vi "_attribute_write_none.vi"(5 "Repeated Capability":string, 7 "Attribute":T1={"Identifier"="", "Descriptive Name"="", "Data Type"=enum."Integer 32", "Command"="", "Access"=enum."Read/Write", "Range Table"="", "Read Callback"="", "Write Callback"="", "Supported Models"="", "Instrument Options"="", "Index"=0, "OPC Wait"=FALSE, "No Status Check"=FALSE, "Cache Only"=FALSE}, 8 "error in":errorcluster caption="error in (no error)", 11 "VISA resource name":refnum<visa-resource-name>) -> (0 "error out":errorcluster, 3 "VISA resource name out":refnum<visa-resource-name>)   [LabVIEW 2020, in "Rohde&Schwarz RTx Oscilloscopes.lvlib" / "rsidr_core.lvlib"]
uses:
  rsidr_core.lvlib
  type_Attribute.ctl
  type_Attribute_Data_Type.ctl
  type_ReadWriteAccess.ctl
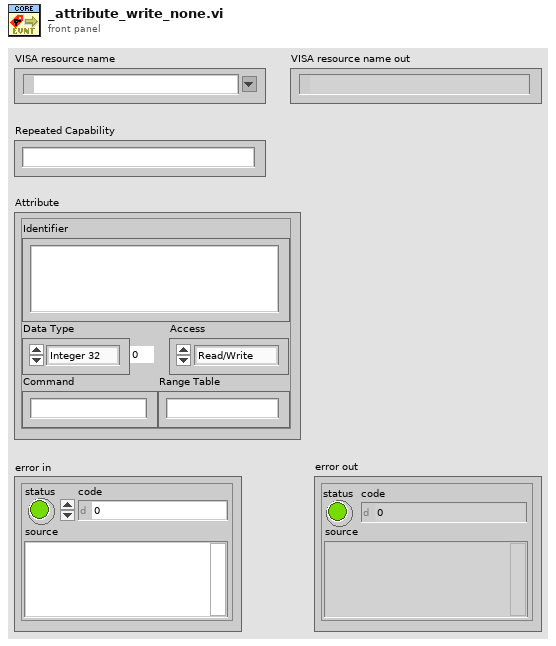
[diagram p1: front panel]
types:
  T1 = typedef "Rohde&Schwarz RTx Oscilloscopes.lvlib/rsidr_core.lvlib/type_Attribute.ctl" = cluster{"Identifier":string, "Descriptive Name":string, "Data Type":T2, "Command":string, "Access":T3, "Range Table":string, "Read Callback":string, "Write Callback":string, "Supported Models":string, "Instrument Options":string, "Index":i32, "OPC Wait":bool, "No Status Check":bool, "Cache Only":bool}
  T2 = typedef "Rohde&Schwarz RTx Oscilloscopes.lvlib/rsidr_core.lvlib/type_Attribute_Data_Type.ctl" = enum16{"Integer 32", "Double", "String", "Boolean", "None", "Integer 64", "RawString"}
  T3 = typedef "Rohde&Schwarz RTx Oscilloscopes.lvlib/rsidr_core.lvlib/type_ReadWriteAccess.ctl" = enum16{"Read Only", "Write Only", "Read/Write"}
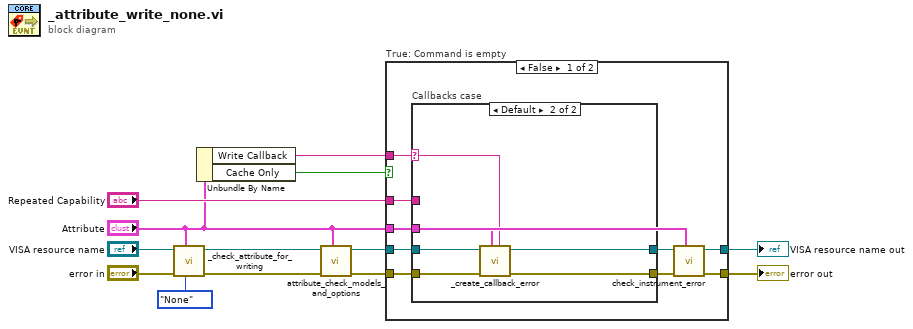
[diagram p0: block diagram]
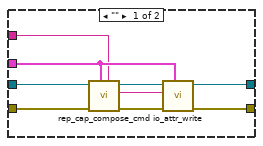
[diagram p2: hidden frame]
diagram:
  n1 = call "_check_attribute_for_writing.vi"("Expected Data Type"=type_Attribute_Data_Type."None" ("Data Type"), "Attribute"="Attribute", "error in"="error in", "VISA resource name"="VISA resource name") -> ("error out"=w8:errorcluster, "VISA resource name out"=w7:refnum<visa-resource-name>)  [unwired: 6 in]
  n2 = Unbundle By Name("Attribute") -> ("Write Callback"=w10:string, "Cache Only"=w1:bool)
  n3 = call "attribute_check_models_and_options.vi"("Attribute"="Attribute", "error in"=w8, "VISA resource name"=w7) -> ("error out"=w6:errorcluster, "VISA resource name out"=w5:refnum<visa-resource-name>)  [unwired: 6 in, 1 out]
  n4 = case "True: Command is empty" shown="False" w1 {
    tunnel: "Repeated Capability" -> [w22 _]
    tunnel: w6 -> [w21 w38]
    tunnel: w5 -> [w20 w39]
    tunnel: "Attribute" -> [w14 _]
    tunnel: [w15 w39] -> w2
    tunnel: [w16 w38] -> w3
    tunnel: w10 -> [w19 _]
    frame False {
      n5 = case "Callbacks case" shown="Default" w19 {
        selector: w19 -> [_ w32]
        tunnel: w20 -> [w30 w36]
        tunnel: w21 -> [w28 w37]
        tunnel: w22 -> [w23 _]
        tunnel: [w27 w34] -> w17
        tunnel: [w26 w35] -> w18
        tunnel: w14 -> [w24 w33]
        frame "" {
          n6 = call "rep_cap_compose_cmd.vi"("Repeated Capability"=w23, "Attribute"=w24, "error in"=w28, "VISA resource name"=w30) -> ("error out"=w29:errorcluster, "Command out"=w25:string, "VISA resource name out"=w31:refnum<visa-resource-name>)  [unwired: 5 in]
          n7 = call "io_attr_write.vi"("Attribute"=w24, "error in"=w29, "write buffer"=w25, "VISA resource name"=w31) -> ("error out"=w26:errorcluster, "VISA resource name out"=w27:refnum<visa-resource-name>)  [unwired: 6 in]
        }
        frame Default {
          n8 = call "_create_callback_error.vi"("Callback Name"=w32, "Attribute"=w33, "error in"=w37, "VISA resource name"=w36) -> ("error out"=w35:errorcluster, "VISA resource name out"=w34:refnum<visa-resource-name>)  [unwired: 6 in]
        }
      }
      n9 = call "check_instrument_error.vi"("Attribute"=w14, "error in"=w18, "VISA resource name"=w17) -> ("error out"=w16:errorcluster, "VISA resource name out"=w15:refnum<visa-resource-name>)  [unwired: 7 in]
    }
    frame True {
    }
  }
  "error out" <- w3
  "VISA resource name out" <- w2
